vi "03.Evd.2_Ask.3.vi"() -> ()   [LabVIEW 2025]
panel:
  in  "Start/stop":bool=TRUE
  out "Tank height (m)":dbl
  in  "R (Radius in m)":dbl=1.0
  in  "V (Volume in L)":dbl=10000.0
  out "Tank":dbl(slide) scale=0.0..100.0
  # "Theoretical calculation of the height of a cylindrical liquid fuel tank"
  # "誓誓誓誓誓"
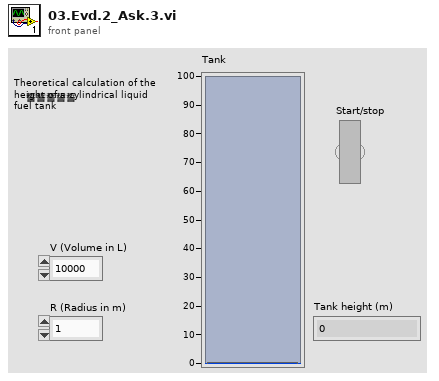
[diagram p1: front panel]
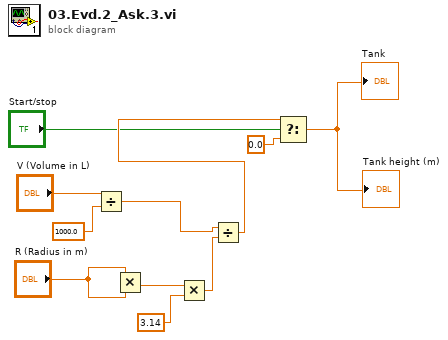
[diagram p0: block diagram]
diagram:
  n1 = Divide(x="V (Volume in L)", y=1000.0) -> (x/y=w1:dbl)
  n2 = Multiply(x="R (Radius in m)", y="R (Radius in m)") -> (x*y=w9:dbl)
  n3 = Multiply(x=w9, y=3.14) -> (x*y=w7:dbl)
  n4 = Divide(x=w1, y=w7) -> (x/y=w6:dbl)
  n5 = Select(t=w6, s="Start/stop", f=0.0 ("y")) -> (s? t:f=→"Tank" →"Tank height (m)":dbl)
